vi "checkForceErrorInRange_old.vi"(8 "error in (no error)":errorcluster, 11 "Model in":refnum<class "Model.lvclass">) -> (0 "error out":errorcluster, 2 "inRangeIsTrue":bool, 3 "Model out":refnum<class "Model.lvclass">)   [LabVIEW 2015]
uses:
  Model.lvclass
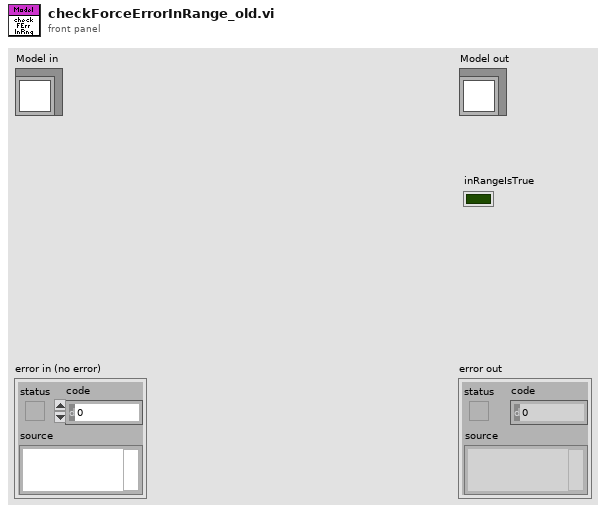
[diagram p1: front panel]
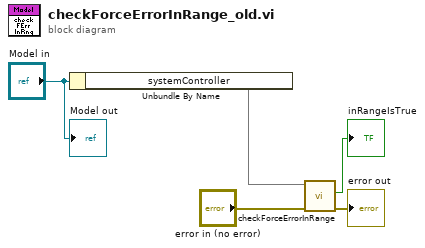
[diagram p0: block diagram]
diagram:
  n1 = Unbundle By Name("Model in") -> ("systemController"=w5)
  n2 = call "checkForceErrorInRange.vi"("error in (no error)"="error in (no error)", "SystemController in"=w5) -> ("error out"=→"error out":errorcluster, "forceErrorInRangeIsTrue"=→"inRangeIsTrue":bool)  [unwired: 7 in, 1 out]
  "Model out" <- "Model in"
